vi "RSMA Receiver -  3 SC 2 Channels.vi"() -> ()   [LabVIEW 2022 SP3]
panel:
  out "SC Bits 2":i8[](array[numeric])
  out "Decoded Message - CH0":string
  out "Constellation Map":cluster{"Constellation":cdb[]}[](graph)
  in  "Tab Control":enum32{"USRP Parameters", "Rx Info", "BER"}(tab)
  in  "USRP ControledParameters":T1={"Active Antenna"="RX2", "Gain (dB)"=0.0, "Carrier Frequency"=2400000000.0, "IQ Rate"=2000000.0, "Active channels"="0,1"} {"IQ Rate" format="%#_6p"; "Carrier Frequency" format="%#_6p"; "Gain (dB)" format="%#_6f"}
  in  "Device selection":refnum<k15>="RIO0"
  in  "Trigger level":dbl=0.01 format="%f"
  out "CH0":T2
  out "CH1":T2
  out "SIG valid? - CH1":bool
  out "SIG valid? - CH0":bool
  out "Frequency offset - CH1":dbl
  out "Frequency offset - CH0":dbl
  out "Coerced Parameters":T3={"IQ Rate"=100000.0, "Carrier  Freq."=100000.0, "Gain"=0.0} {"Gain" format="%#_6f"; "Carrier  Freq." format="%#_6p"; "IQ Rate" format="%#_6p"}
  out "Error out":errorcluster
  out "Acc. BER - CH1":dbl format="%#_4g"
  in  "Refresh Button":bool
  in  "Record BER":bool
  in  "Expected message - CH0":string="Lorem ipsum dolor sit amet, consetetur sadipscing elitr, sed diam nonumy eirmod tempor invidunt ut labore et dolore magna aliquyam erat, sed diam volu"
  in  "Expected message - CH1":string="ptua. At vero eos et accusam et justo duo dolores et ea rebum. Stet clita kasd gubergren, no sea takimata sanctus est Lorem ipsum dolor sit amet. Lore"
  out "Acum. Err - CH0":dbl
  out "Acum. Err - CH1":dbl
  out "No. Bits - CH0":dbl format="%#_6f"
  out "No. Bits - CH1":dbl
  out "Inst. BER - CH0":dbl format="%#_4g"
  out "Inst. BER - CH1":dbl format="%#_4g"
  out "Acc. BER - CH0":dbl format="%#_4g"
  in  "error in (no error)":errorcluster
  out "Decoded message - CH1":string
  # "RSMA Receiver"
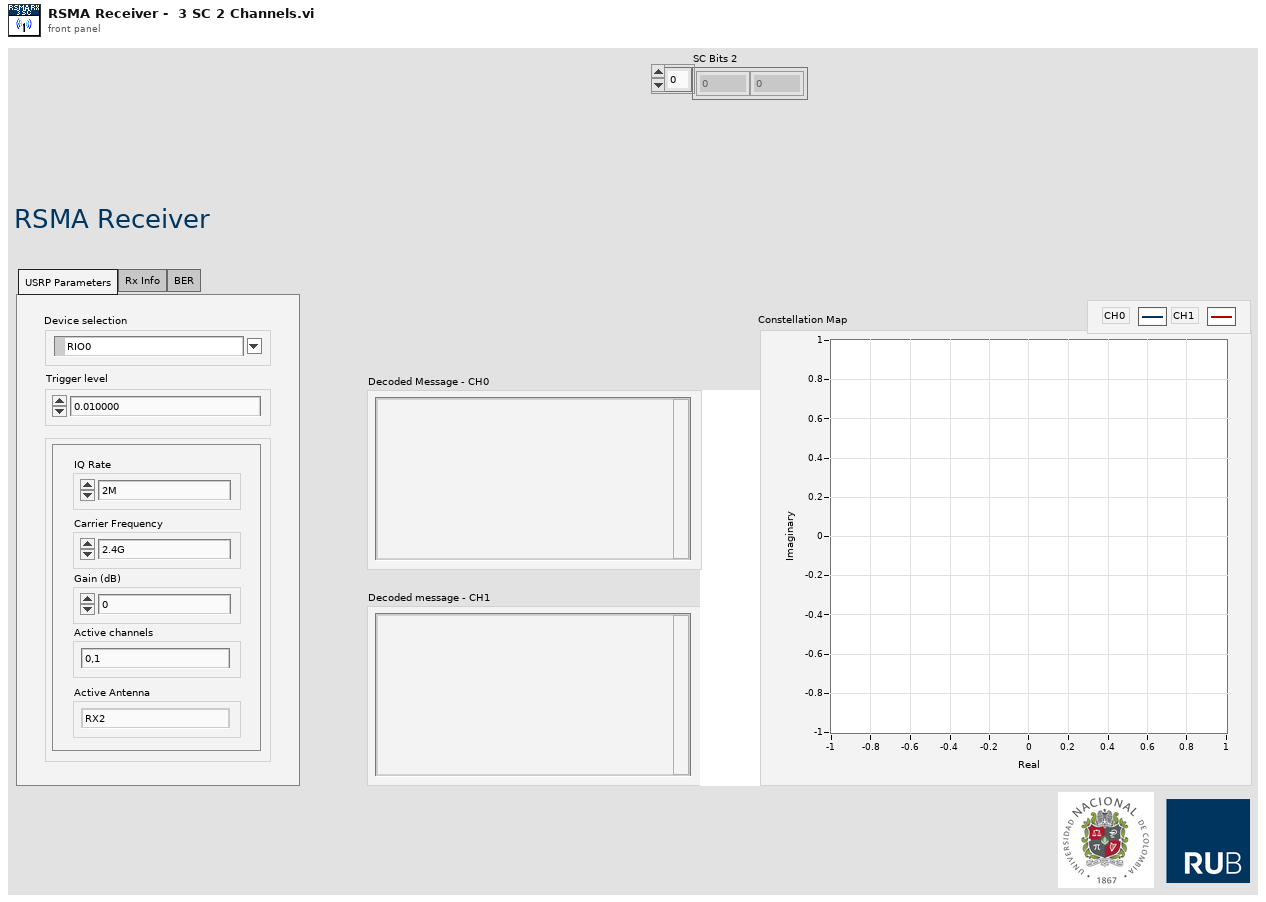
[diagram p1: front panel]
types:
  T1 = cluster{"Active Antenna":string, "Gain (dB)":dbl, "Carrier Frequency":dbl, "IQ Rate":dbl, "Active channels":string}
  T2 = cluster{"Modulation type":enum16{"QPSK(4QAM)", "64QAM", "16QAM", "BPSK"}, "BCC rate (k/n)":enum16{"1/2", "2/3", "3/4"}}
  T3 = cluster{"IQ Rate":dbl, "Carrier  Freq.":dbl, "Gain":dbl}
  T4 = cluster{"coerced IQ rate":dbl, "coerced carrier frequency":dbl, "coerced gain":dbl}
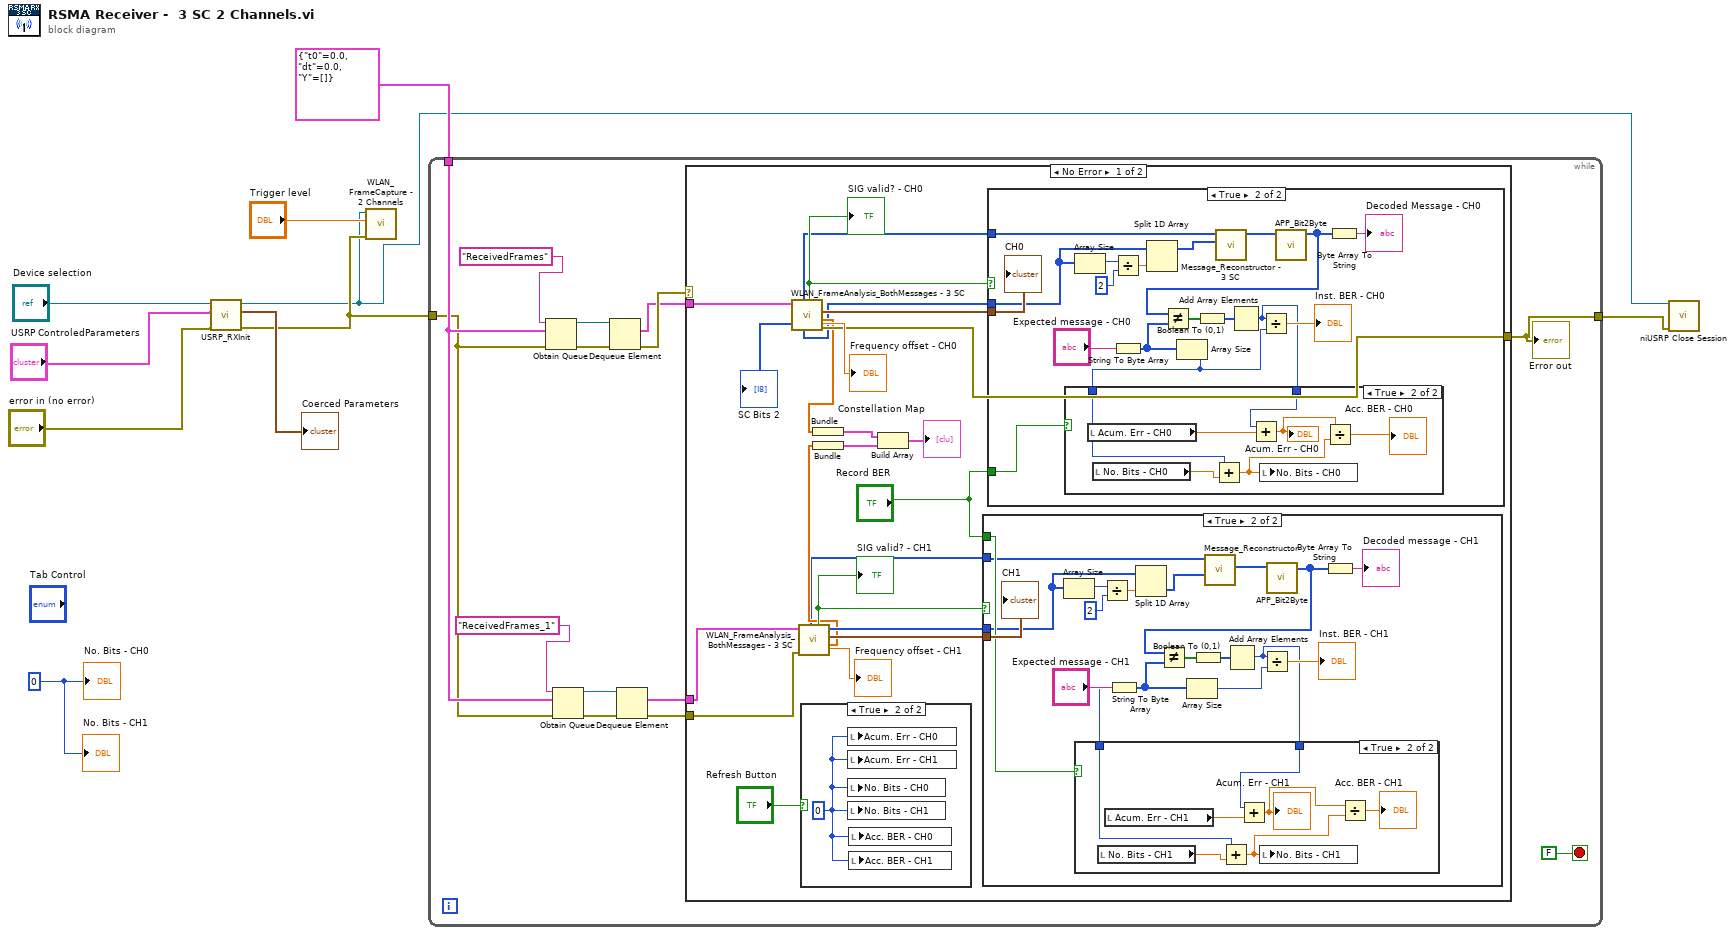
[diagram p0: block diagram]
diagram:
  w1 = 0
  n1 = call "USRP_RXInit.vi"("device names"="Device selection", "USRP ControledParameters"="USRP ControledParameters", "error in (no error)"="error in (no error)") -> ("session handle out"=w4:refnum<k15>, "USRP CoercedParamters"=→"Coerced Parameters":T4, "error out"=w8:errorcluster)  [unwired: 5 in]
  n2 = call "WLAN_FrameCapture - 2 Channels.vi"("error in (no error)"=w8, "Trigger level"="Trigger level", "session handle"=w4) -> ()  [unwired: 8 in]
  n3 = while {
    tunnel: w8 -> [w14]
    tunnel: cluster{"t0":dbl, "dt":dbl, "Y":cdb[]} {"t0"=0.0, "dt"=0.0, "Y"=[]} ("data") -> [w15]
    tunnel: [w19] -> w5
    stop <- FALSE stop-if-true
    n4 = Obtain Queue(name (unnamed)="ReceivedFrames", element data type=w15, error in (no error)=w14) -> (queue out=w24:refnum<queue>, error out=w21:errorcluster)  [unwired: 2 in, 1 out]
    n5 = Obtain Queue(name (unnamed)="ReceivedFrames_1", element data type=w15, error in (no error)=w14) -> (queue out=w18:refnum<queue>, error out=w17:errorcluster)  [unwired: 2 in, 1 out]
    n6 = Dequeue Element(queue=w24, error in (no error)=w21) -> (element=w22:cluster{"t0":dbl, "dt":dbl, "Y":cdb[]}, error out=w23:errorcluster)  [unwired: 1 in, 2 out]
    n7 = Dequeue Element(queue=w18, error in (no error)=w17) -> (element=w12:cluster{"t0":dbl, "dt":dbl, "Y":cdb[]}, error out=w13:errorcluster)  [unwired: 1 in, 2 out]
    n8 = case shown="No Error" w23 {
      selector: w23 -> [_ w97]
      tunnel: w22 -> [w41 _]
      tunnel: [w42 w97] -> w19
      tunnel: w13 -> [w36 _]
      tunnel: w12 -> [w35 _]
      frame No Error {
        n9 = call "WLAN_FrameAnalysis_BothMessages - 3 SC.vi"("input cluster"=w41) -> ("error out"=w42:errorcluster, "Constellation"=w34:cdb[], "Modulation parameter"=w43:T2, "Frequency offset"=→"Frequency offset - CH0":dbl, "SIG valid?"=w44:bool, "SC Bits 2"=w25:i8[], "Base Bits"=w27:i8[])  [unwired: 3 in, 1 out]
        "SIG valid? - CH0" <- w44
        "SC Bits 2" <- w25
        n10 = call "WLAN_FrameAnalysis_BothMessages - 3 SC.vi"("error in (no error)"=w36, "input cluster"=w35) -> ("Constellation"=w33:cdb[], "Modulation parameter"=w37:T2, "SC Bits"=w38:i8[], "Frequency offset"=→"Frequency offset - CH1":dbl, "SIG valid?"=w39:bool, "Base Bits"=w26:i8[])  [unwired: 2 in, 2 out]
        "SIG valid? - CH1" <- w39
        n11 = case shown="True" "Refresh Button" {
          frame False {
          }
          frame True {
            w46 = 0
            n12 = local write "Acum. Err - CH0"(w46) -> ()
            n13 = local write "Acum. Err - CH1"(w46) -> ()
            n14 = local write "No. Bits - CH0"(w46) -> ()
            n15 = local write "No. Bits - CH1"(w46) -> ()
            n16 = local write "Acc. BER - CH0"(w46) -> ()
            n17 = local write "Acc. BER - CH1"(w46) -> ()
          }
        }
        n18 = Bundle("Constellation"=w34) -> (w30:cluster{"Constellation":cdb[]})  [unwired: 1 in]
        n19 = Bundle("Constellation"=w33) -> (w31:cluster{"Constellation":cdb[]})  [unwired: 1 in]
        n20 = Build Array(w30, w31) -> (→"Constellation Map":cluster{"Constellation":cdb[]}[])
        n21 = case shown="True" w39 {
          tunnel: w38 -> [_ w49]
          tunnel: w37 -> [_ w64]
          tunnel: "Record BER" -> [_ w59]
          tunnel: w26 -> [_ w51]
          frame False {
          }
          frame True {
            n22 = Array Size(array=w49) -> (size(s)=w53:i32)
            n23 = Divide(x=w53, y=2) -> (x/y=w54:dbl)
            n24 = String To Byte Array(string="Expected message - CH1") -> (unsigned byte array=w57:u8[])
            n25 = Split 1D Array(array=w49, index=w54) -> (second subarray=w50:i8[])  [unwired: 1 out]
            n26 = Array Size(array=w57) -> (size(s)=w56:i32)
            n27 = call "Message_Reconstructor.vi"("Wp2"=w50, "Wc"=w51) -> ("W2"=w48:u8[])  [unwired: 8 in, 1 out]
            n28 = call "APP_Bit2Byte.vi"("input bit stream"=w48) -> ("output byte stream"=w47:u8[])  [unwired: 10 in]
            n29 = Not Equal?(x=w47, y=w57) -> (x != y?=w61:bool[])
            n30 = Boolean To (0,1)(Boolean=w61) -> (0, 1=w62:i16[])
            n31 = Add Array Elements(numeric array=w62) -> (sum=w55:i16)
            n32 = case shown="True" w59 {
              tunnel: w56 -> [_ w70]
              tunnel: w55 -> [_ w68]
              frame False {
              }
              frame True {
                n33 = local read "No. Bits - CH1"() -> (w71:dbl)
                n34 = local read "Acum. Err - CH1"() -> (w69:dbl)
                n35 = Add(x=w70, y=w71) -> (x+y=w67:dbl)
                n36 = Add(x=w68, y=w69) -> (x+y=w66:dbl)
                "Acum. Err - CH1" <- w66
                n37 = local write "No. Bits - CH1"(w67) -> ()
                n38 = Divide(x=w66, y=w67) -> (x/y=→"Acc. BER - CH1":dbl)
              }
            }
            n39 = Divide(x=w55, y=w56) -> (x/y=→"Inst. BER - CH1":dbl)
            n40 = Byte Array To String(unsigned byte array=w47) -> (string=→"Decoded message - CH1":string)
            "CH1" <- w64
          }
        }
        n41 = case shown="True" w44 {
          tunnel: w25 -> [_ w75]
          tunnel: w43 -> [_ w89]
          tunnel: "Record BER" -> [_ w85]
          tunnel: w27 -> [_ w74]
          frame False {
          }
          frame True {
            n42 = Array Size(array=w75) -> (size(s)=w80:i32)
            n43 = Divide(x=w80, y=2) -> (x/y=w78:dbl)
            n44 = String To Byte Array(string="Expected message - CH0") -> (unsigned byte array=w84:u8[])
            n45 = Split 1D Array(array=w75, index=w78) -> (first subarray=w77:i8[])  [unwired: 1 out]
            n46 = Array Size(array=w84) -> (size(s)=w82:i32)
            n47 = call "Message_Reconstructor - 3 SC.vi"("Wp"=w77, "Wc"=w74) -> ("W1"=w73:u8[])  [unwired: 9 in]
            n48 = call "APP_Bit2Byte.vi"("input bit stream"=w73) -> ("output byte stream"=w72:u8[])  [unwired: 10 in]
            n49 = Not Equal?(x=w72, y=w84) -> (x != y?=w87:bool[])
            n50 = Boolean To (0,1)(Boolean=w87) -> (0, 1=w88:i16[])
            n51 = Add Array Elements(numeric array=w88) -> (sum=w81:i16)
            n52 = case shown="True" w85 {
              tunnel: w82 -> [_ w95]
              tunnel: w81 -> [_ w93]
              frame False {
              }
              frame True {
                n53 = local read "Acum. Err - CH0"() -> (w94:dbl)
                n54 = local read "No. Bits - CH0"() -> (w96:dbl)
                n55 = Add(x=w95, y=w96) -> (x+y=w92:dbl)
                n56 = Add(x=w93, y=w94) -> (x+y=w91:dbl)
                "Acum. Err - CH0" <- w91
                n57 = local write "No. Bits - CH0"(w92) -> ()
                n58 = Divide(x=w91, y=w92) -> (x/y=→"Acc. BER - CH0":dbl)
              }
            }
            n59 = Divide(x=w81, y=w82) -> (x/y=→"Inst. BER - CH0":dbl)
            n60 = Byte Array To String(unsigned byte array=w72) -> (string=→"Decoded Message - CH0":string)
            "CH0" <- w89
          }
        }
      }
      frame Error {
      }
    }
    "Error out" <- w19
  }
  n61 = call <instrlib>:"niUSRP Close Session.vi"("session handle"=w4, "error in (no error)"=w5) -> ()  [unwired: 13 in, 1 out]
  "No. Bits - CH0" <- w1
  "No. Bits - CH1" <- w1
